vi "Bodies_DH_update.vi"(8 "error in (no error)":errorcluster, 10 "JointValues(rad)":dbl[](array[numeric]) format="%.2f", 11 "Body.lvclass In":refnum<class "Bodies.lvclass">) -> (0 "error out":errorcluster, 3 "Body.lvclass Out":refnum<class "Bodies.lvclass">)   [LabVIEW 2015, in "Bodies.lvclass"]
uses:
  Bodies.lvclass
  <vilib>/Analysis/Matrix/Datatypes/RealMatrix.ctl
  Bodies.lvclass/Bodies.ctl
  <vilib>/Analysis/BLAS.llb/LV_Transpose.ctl
  <vilib>/Analysis/BLAS.llb/dgemm - General Matrix-Matrix Product (DBL).vi
  <vilib>/Analysis/Matrix/NI_Matrix.lvlib
  <vilib>/gmath/NI_Gmath.lvlib
  <vilib>/Analysis/NI_AALBLAS.lvlib
panel:
  out "T_0":dbl[][][](array[numeric]) format="%4_4f"
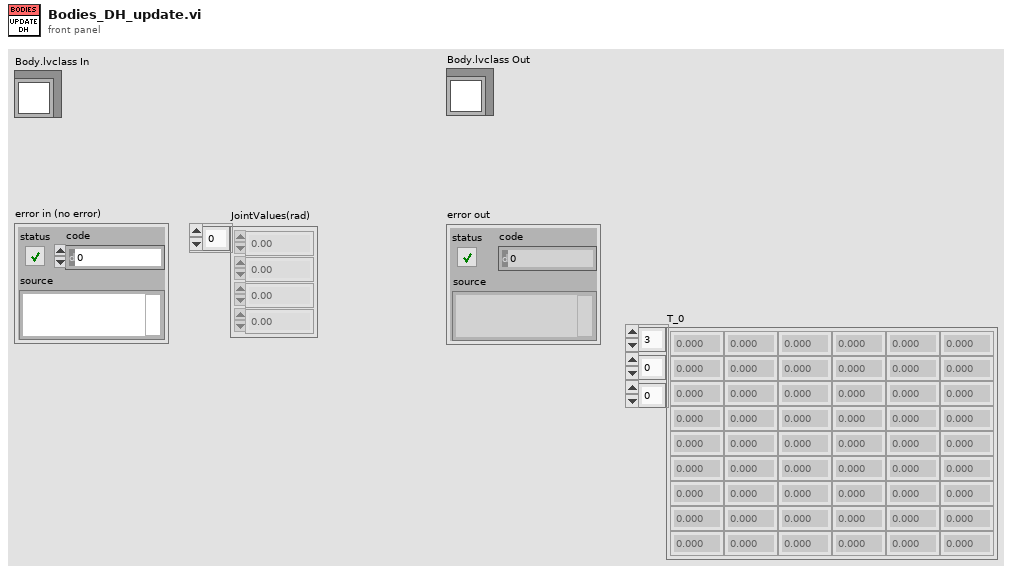
[diagram p1: front panel]
types:
  T1 = typedef "NI_Matrix.lvlib/RealMatrix.ctl" = dbl[][]
  T2 = cluster{"Y Values":dbl[][], "Tables":i32[][][], "Variables input decode":i32[], "Variables output decode":i32[]}[]
  T3 = typedef "NI_AALBLAS.lvlib/LV_Transpose.ctl" = i32
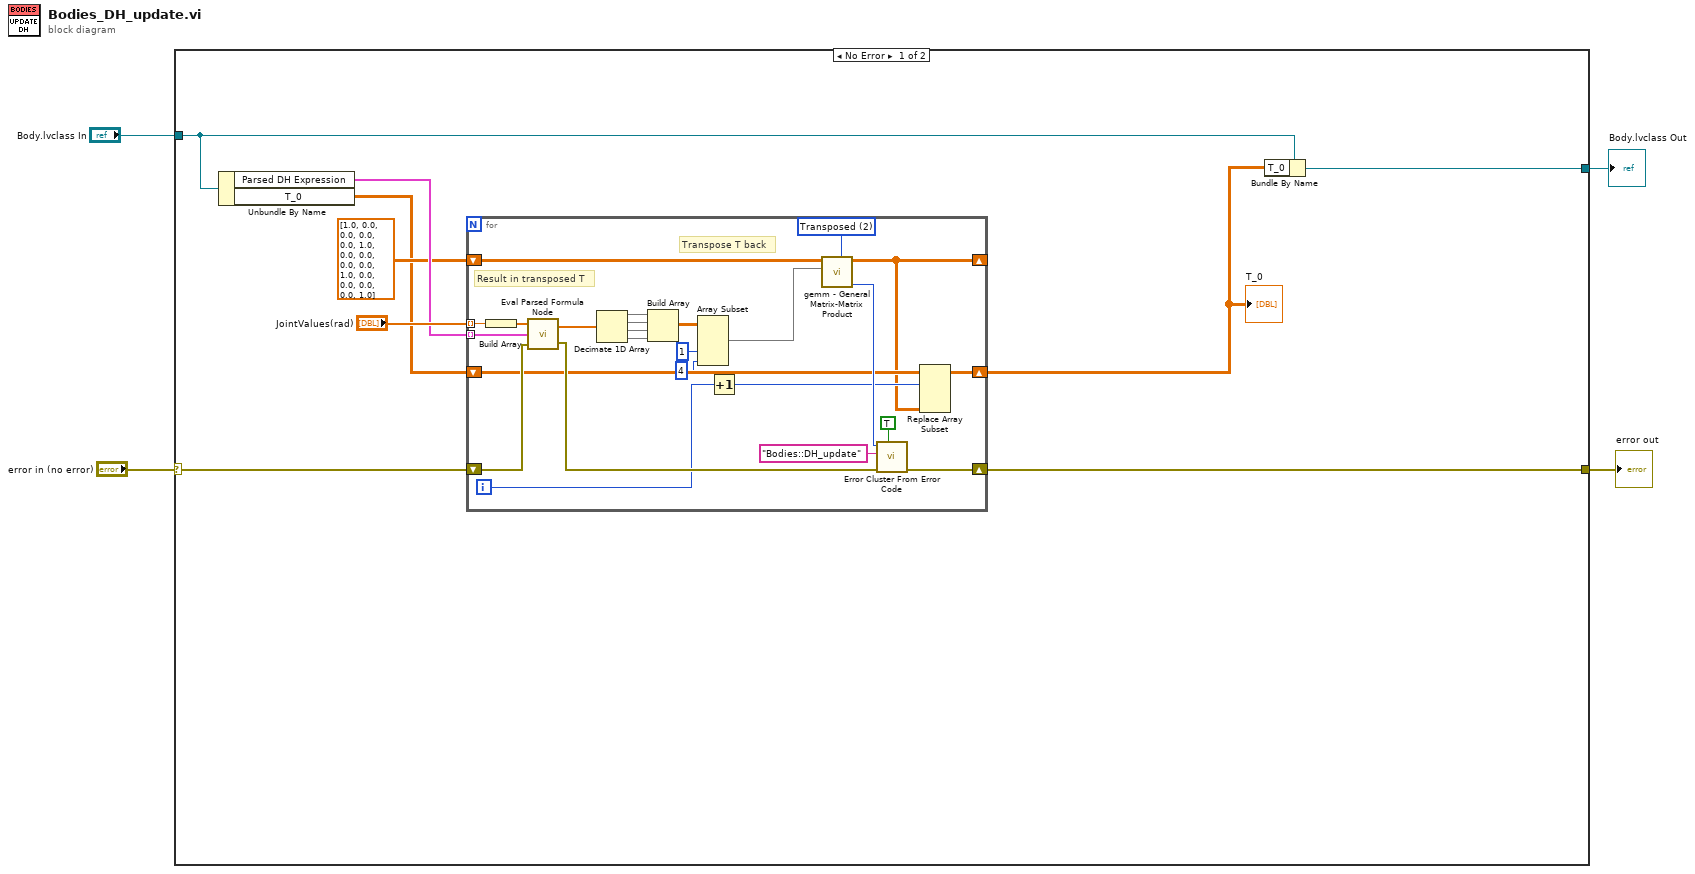
[diagram p0: block diagram]
diagram:
  n1 = case shown="No Error" "error in (no error)" {
    selector: "error in (no error)" -> [w11 w40]
    tunnel: "Body.lvclass In" -> [w13 w39]
    tunnel: [w12 w39] -> w2
    tunnel: [w10 w40] -> w1
    frame No Error {
      n2 = Unbundle By Name(w13) -> ("Parsed DH Expression"=w8:T2, "T_0"=w6:dbl[][][])
      n3 = for {
        tunnel: w8 -> [w34] mode=indexing
        tunnel: "JointValues(rad)" -> [w37] mode=indexing
        shift-right: [w31] -> w10
        shift-left: w11 -> [w36]
        shift-right: [w21] -> _
        shift-left: T1 [[1.0, 0.0, 0.0, 0.0], [0.0, 1.0, 0.0, 0.0], [0.0, 0.0, 1.0, 0.0], [0.0, 0.0, 0.0, 1.0]] ("Real Matrix") -> [w35]
        shift-right: [w20] -> w5
        shift-left: w6 -> [w24]
        i -> [w23]
        w19 = T3 2 items=["Direct", "Conjugated & Transposed", "Transposed"] ("operation B")
        # "Transpose T back"
        # "Result in transposed T"
        n4 = Build Array(w37) -> (w38:dbl[])
        n5 = call <vilib>:"Eval Parsed Formula Node.vi"("error in (no error)"=w36, "Parsed Formula Node"=w34, "Input Values"=w38) -> ("error out"=w32:errorcluster, "Output Values"=w15:dbl[])
        n6 = Decimate 1D Array(w15) -> (w25:dbl[], w26:dbl[], w27:dbl[], w28:dbl[])
        n7 = Build Array(w25, w26, w27, w28) -> (w18:dbl[][])
        n8 = Array Subset(array=w18, index (col)=1 ("index"), length (col)=4 ("length")) -> (w14:dbl[][])  [unwired: 2 in]
        n9 = Increment(x=w23) -> (x+1=w22:i32)
        n10 = call-poly <vilib>:"gemm - General Matrix-Matrix Product.vi"("operation B"=w19, "B"=w14, "A"=w35) -> ("error"=w33:i32, "dgemm"=w21:T1)  [unwired: 7 in]
        n11 = call <vilib>:"Error Cluster From Error Code.vi"("show call chain? (False)"=TRUE, "error in (no error)"=w32, "error message (\"\")"="Bodies::DH_update" ("error message (\"\")"), "error code (0)"=w33) -> ("error out"=w31:errorcluster)  [unwired: 5 in]
        n12 = Replace Array Subset(array=w24, new element=w21, index (dim 0)=w22) -> (w20:dbl[][][])  [unwired: 2 in]
      }
      "T_0" <- w5
      n13 = Bundle By Name(cluster=w13, "T_0"=w5) -> (w12:refnum<class "Bodies.lvclass">)
    }
    frame Error {
    }
  }
  "Body.lvclass Out" <- w2
  "error out" <- w1
